vi "ReducedSample.vi"() -> ()   [LabVIEW 2019]
uses:
  <vilib>/express/express controls/BuildTableBlock.llb/mergeTable.vi/Instance           1 18Saved   mergeTable .vi
panel:
  in  "Enable 2":bool=TRUE caption="Enable"
  out "Table":string[][](table)
  in  "stop":bool
  out "Sine":dynamicdata(graph)
  in  "Enable":bool=TRUE
  out "Mean":dbl
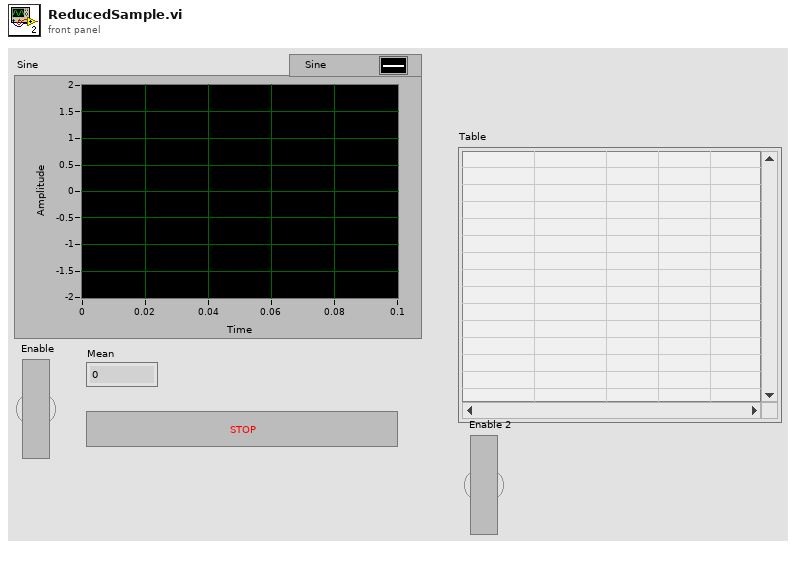
[diagram p1: front panel]
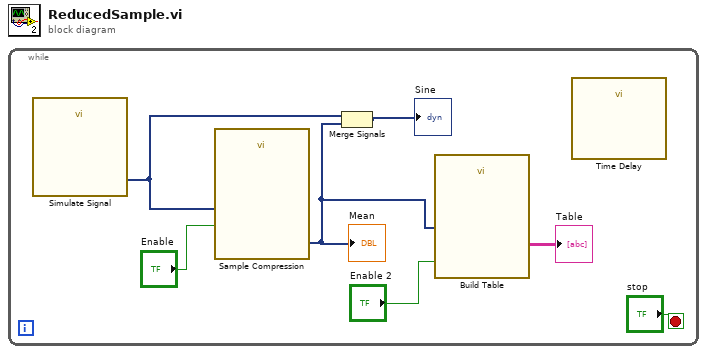
[diagram p0: block diagram]
diagram:
  n1 = while {
    stop <- "stop" stop-if-true
    n2 = call "Simulate Signal"() -> ("Sine"=w6:dynamicdata)  [unwired: 14 in, 1 out]
    n3 = call "Sample Compression"("Enable"="Enable", "Signals"=w6) -> ("Mean"=w2:dynamicdata)  [unwired: 7 in, 2 out]
    "Mean" <- w2
    n4 = Merge Signals(w6, w2) -> (→"Sine":dynamicdata)
    n5 = call "Build Table"("Enable"="Enable 2", "Signals"=w2) -> ("Table"=→"Table":string[][])  [unwired: 3 in, 6 out]
    n6 = call "Time Delay"() -> ()  [unwired: 11 in, 1 out]
  }
